vi "LITVC Shift Variables.vi"(8 "error in":errorcluster) -> (0 "error out":errorcluster, 3 "VARS FFT_DAS":T1={"queue data"={"Command"="", "Variant Data"=variant}, "error"={"status"=FALSE, "code"=0, "source"=""}, "FFT_DAS queue"=refnum, "Q_TO"=0, "WDT_TO"=0.0, "LogErrors?"=FALSE, "Main.ini Ref"=refnum, "Connected? 1"=FALSE, "Address 1"="", "Link_Name"="", "Config Vars"={"Distance/Count"=4.5, "samples/ch"=50, "Task_TO"=10.0, "Kc"=-0.32, "B"=1.46}, "DataFilePath"=path "", "Calibrate"=FALSE, "Cal_Slope-Offset"=[], "TestTable"=[], "Test Status"=enum."Idle", "Parameter Table Out"=[], "Test Start Time"="", "Test Stop Time"="", "Test Timing Mode"=enum."Semi-Automatic", "Number of sensors"=0.0} {"Config Vars"."B" format="%0.2f"; "Config Vars"."Kc" format="%0.2f"; "Config Vars"."Distance/Count" format="%0.2f"; "Config Vars"."samples/ch" min=0 max=-1048576; "Config Vars"."Task_TO" format="%0.2f"; "WDT_TO" format="%_4g"})   [LabVIEW 2018]
uses:
  Controls/FFT_DAS Shift Variables.ctl
  COMM_Queues/Command Queue Cluster.ctl
  COMM_Queues/Command_Queue_Ref.ctl
  WRIS_Config Vars Cluster.ctl
  Controls/Timing Mode.ctl
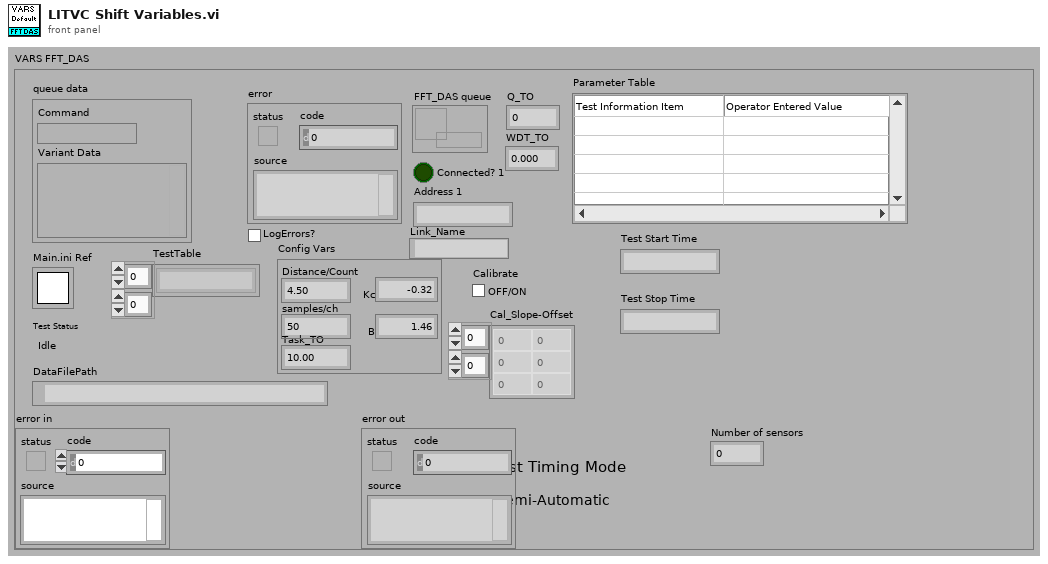
[diagram p1: front panel]
types:
  T1 = typedef "FFT_DAS Shift Variables.ctl" = cluster{"queue data":T2, "error":errorcluster, "FFT_DAS queue":T3, "Q_TO":i32, "WDT_TO":dbl, "LogErrors?":bool, "Main.ini Ref":refnum<k1>, "Connected? 1":bool, "Address 1":string, "Link_Name":string, "Config Vars":T4, "DataFilePath":path, "Calibrate":bool, "Cal_Slope-Offset":dbl[][], "TestTable":string[][], "Test Status":enum16{"Idle", "Test Running", "Test Paused", "Test Completed"}, "Parameter Table Out":string[][], "Test Start Time":string, "Test Stop Time":string, "Test Timing Mode":T5, "Number of sensors":dbl}
  T2 = typedef "Command Queue Cluster.ctl" = cluster{"Command":string, "Variant Data":variant}
  T3 = typedef "Command_Queue_Ref.ctl" = refnum<queue>
  T4 = typedef "WRIS_Config Vars Cluster.ctl" = cluster{"Distance/Count":dbl, "samples/ch":i32, "Task_TO":dbl, "Kc":dbl, "B":dbl}
  T5 = typedef "Timing Mode.ctl" = enum16{"Manual", "Automatic", "Semi-Automatic"}
  T6 = enum16{"Idle", "Test Running", "Test Paused", "Test Completed"}
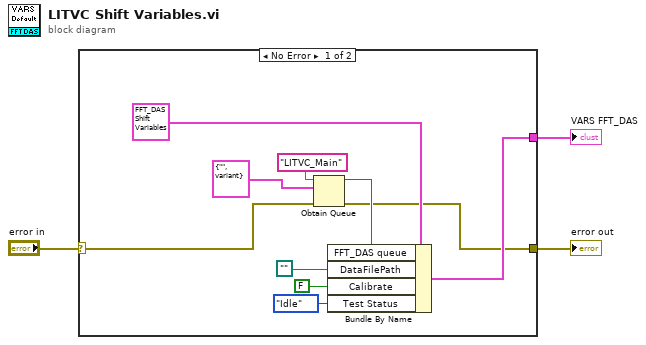
[diagram p0: block diagram]
diagram:
  n1 = case shown="No Error" "error in" {
    selector: "error in" -> [w7 w14]
    tunnel: [w13 _] -> w3
    tunnel: [w6 w14] -> w1
    frame No Error {
      n2 = Obtain Queue(name (unnamed)="LITVC_Main", element data type=T2 {"Command"="", "Variant Data"=variant} ("queue data"), error in (no error)=w7) -> (queue out=w9:refnum<queue>, error out=w6:errorcluster)  [unwired: 2 in, 1 out]
      n3 = Bundle By Name(cluster=T1 {"queue data"={"Command"="", "Variant Data"=variant}, "error"={"status"=FALSE, "code"=0, "source"=""}, "FFT_DAS queue"=refnum, "Q_TO"=0, "WDT_TO"=0.0, "LogErrors?"=FALSE, "Main.ini Ref"=refnum, "Connected? 1"=FALSE, "Address 1"="", "Link_Name"="", "Config Vars"={"Distance/Count"=0.0, "samples/ch"=0, "Task_TO"=0.0, "Kc"=0.0, "B"=0.0}, "DataFilePath"=path "", "Calibrate"=FALSE, "Cal_Slope-Offset"=[], "TestTable"=[], "Test Status"=enum."Idle", "Parameter Table Out"=[], "Test Start Time"="", "Test Stop Time"="", "Test Timing Mode"=enum."Manual", "Number of sensors"=0.0} ("VARS WRIS"), "FFT_DAS queue"=w9, "DataFilePath"=path "", "Calibrate"=FALSE, "Test Status"=T6."Idle") -> (w13:T1)
    }
    frame Error {
    }
  }
  "VARS FFT_DAS" <- w3
  "error out" <- w1
